vi "Purge Complete.vi"(5 "Purge Time":u32, 6 "Status":string, 7 "Log File Refnum in":refnum<file>, 8 "error in":errorcluster, 9 "UI Data in":T1, 10 "Handshake Notifier in":refnum<notifier>, 11 "Message Queues in":T3) -> (0 "error out":errorcluster, 1 "UI Data out":T1, 2 "Handshake Notifier out":refnum<notifier>, 3 "Message Queues out":T3, 4 "Log File Refnum out":refnum<file>)   [LabVIEW 2014, in "Controller.lvlib"]
doc: "After the purge time has elapsed, turn off the primary fan."
uses:
  Controller.lvlib
  controls/MHL UI Data.ctl
  controls/MHL Status.ctl
  support/Message Queue/All Message Queues.ctl
  support/Message Queue/Message Cluster.ctl
  support/Boiler System Globals.vi
  support/Message Queue/Message Queue.lvlib
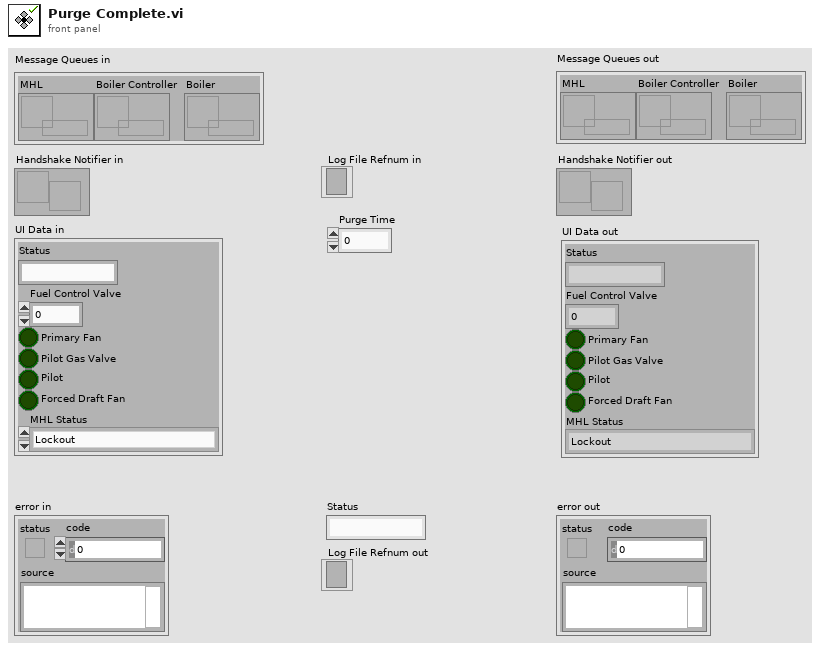
[diagram p1: front panel]
types:
  T1 = typedef "MHL UI Data.ctl" = cluster{"Status":string, "Fuel Control Valve":u32, "Primary Fan":bool, "Pilot Gas Valve":bool, "Pilot":bool, "Forced Draft Fan":bool, "MHL Status":T2}
  T2 = typedef "MHL Status.ctl" = enum16{"Lockout", "Ready", "Pre-Purge", "Pre-Purge Complete", "Pilot On", "Boiler Running", "Shutdown", "Purge"}
  T3 = typedef "Message Queue.lvlib/All Message Queues.ctl" = cluster{"MHL":refnum<queue>, "Boiler Controller":refnum<queue>, "Boiler":refnum<queue>}
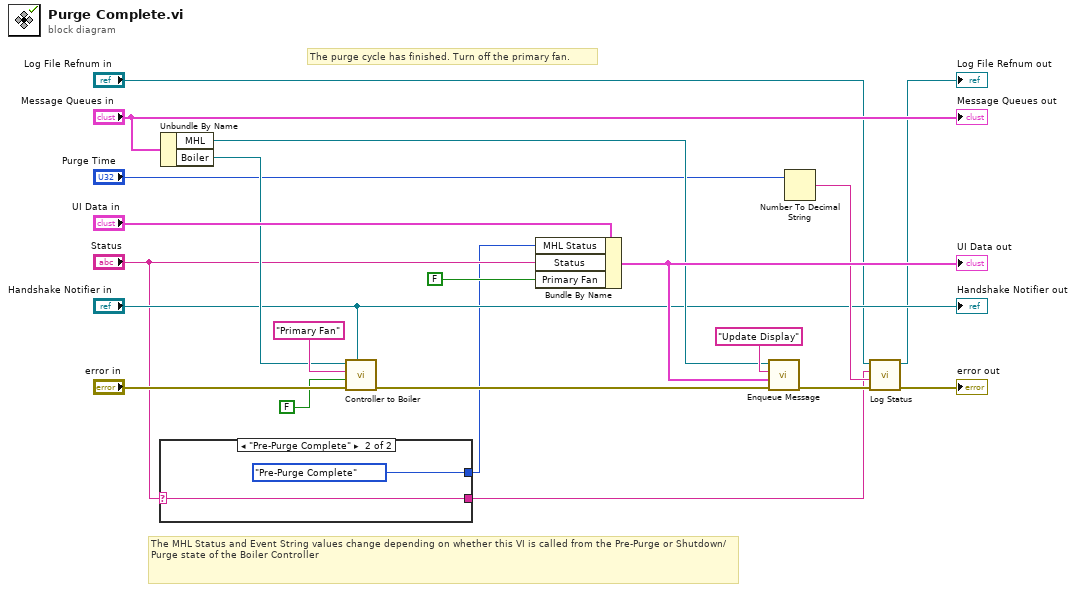
[diagram p0: block diagram]
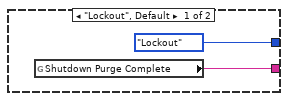
[diagram p2: hidden frame]
diagram:
  # "The MHL Status and Event String values change depending on whether this VI is called from the Pre-Purge or Shutdown/Purge state of the Boiler Controller"
  # "The purge cycle has finished. Turn off the primary fan."
  n1 = case shown="\"Pre-Purge Complete\"" "Status" {
    selector: "Status" -> [_ w25]
    tunnel: [w22 w25] -> w3
    tunnel: [MHL_Status."Lockout" ("MHL Status") MHL_Status."Pre-Purge Complete" ("MHL Status")] -> w4
    frame "Lockout", Default {
      n2 = global read "Boiler System Globals.vi" "Shutdown Purge Complete"() -> (w22:string)
    }
    frame "Pre-Purge Complete" {
    }
  }
  n3 = Unbundle By Name("Message Queues in") -> ("MHL"=w10:refnum<queue>, "Boiler"=w9:refnum<queue>)
  n4 = call "Controller to Boiler.vi"("Notifier"="Handshake Notifier in", "error in"="error in", "Message Data"=FALSE ("Primary Fan"), "Message"="Primary Fan", "Boiler Queue in"=w9) -> ("error out"=w21:errorcluster)  [unwired: 4 in, 2 out]
  n5 = Bundle By Name(cluster="UI Data in", "MHL Status"=w4, "Status"="Status", "Primary Fan"=FALSE) -> (w15:T1)
  "UI Data out" <- w15
  n6 = call "Enqueue Message.vi"("error in (no error)"=w21, "Message Data"=w15, "Message"="Update Display", "Message Queue"=w10) -> ("error out"=w17:errorcluster)  [unwired: 6 in, 1 out]
  n7 = Number To Decimal String(number="Purge Time") -> (decimal integer string=w8:string)  [unwired: 1 in]
  n8 = call "Log Status.vi"("error in"=w17, "Event Data String (-)"=w8, "Event String"=w3, "Log File Refnum In"="Log File Refnum in") -> ("error out"=→"error out":errorcluster, "Log File Refnum Out"=→"Log File Refnum out":refnum<file>)  [unwired: 6 in]
  "Message Queues out" <- "Message Queues in"
  "Handshake Notifier out" <- "Handshake Notifier in"
